vi "get_backlash_compensation.vi"(8 "error in (no error)":errorcluster caption="错误输入（无错误）", 11 "OneMotion输入":refnum<class "OneMotion.lvclass">) -> (0 "error out":errorcluster caption="错误输出", 2 "backlash compensation":dbl, 3 "OneMotion输出":refnum<class "OneMotion.lvclass">)   [LabVIEW 2016, in "MotionControl.lvlib" / "OneMotion.lvclass"]
uses:
  <userlib>/MotionControl/OneMotion/OneMotion.lvclass
  <userlib>/MotionControl/OneMotion/OneMotion.lvclass/OneMotion.ctl
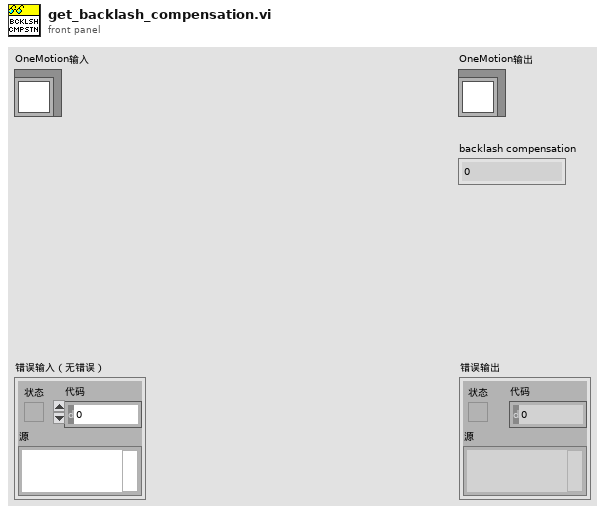
[diagram p1: front panel]
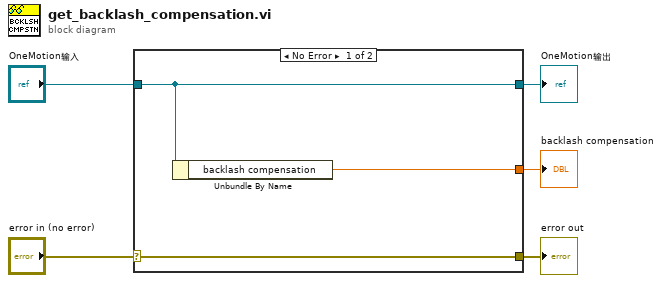
[diagram p0: block diagram]
diagram:
  n1 = case shown="No Error" "error in (no error)" {
    selector: "error in (no error)" -> [w8 w9]
    tunnel: [w8 w9] -> w4
    tunnel: [w7 w10] -> w2
    tunnel: "OneMotion输入" -> [w7 w10]
    tunnel: [w6 _] -> w1
    frame No Error {
      n2 = Unbundle By Name(w7) -> ("backlash compensation"=w6:dbl)
    }
    frame Error {
    }
  }
  "error out" <- w4
  "OneMotion输出" <- w2
  "backlash compensation" <- w1
